vi "Write Next Trace ID.vi"(8 "error in (no error)":errorcluster, 10 "Next Trace ID":u64, 11 "Trace Controller in":refnum<class "Trace Controller.lvclass">) -> (0 "error out":errorcluster, 3 "Trace Controller out":refnum<class "Trace Controller.lvclass">)   [LabVIEW 2014, in "Robot Actor Framework.lvlib" / "Trace.lvlib" / "Trace Controller.lvclass"]
uses:
  Trace Controller.lvclass
  Trace Controller.lvclass/Trace Controller.ctl
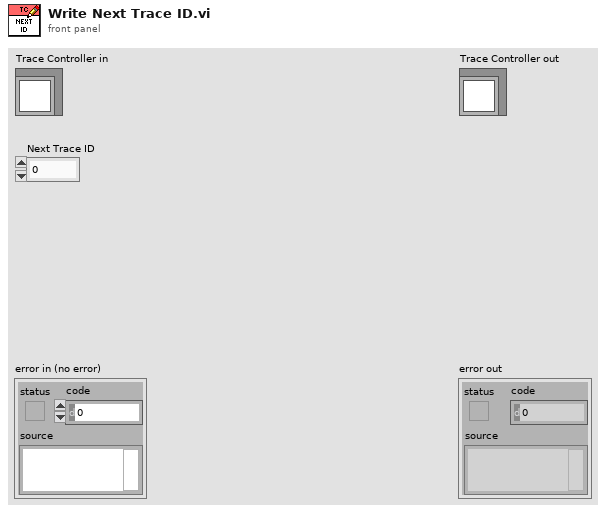
[diagram p1: front panel]
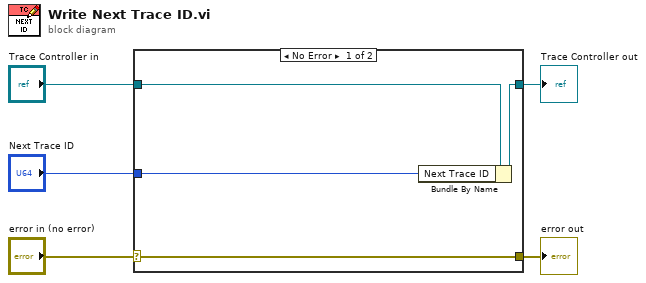
[diagram p0: block diagram]
diagram:
  n1 = case shown="No Error" "error in (no error)" {
    selector: "error in (no error)" -> [w9 w10]
    tunnel: [w9 w10] -> w4
    tunnel: [w7 w11] -> w2
    tunnel: "Trace Controller in" -> [w8 w11]
    tunnel: "Next Trace ID" -> [w6 _]
    frame No Error {
      n2 = Bundle By Name(cluster=w8, "Next Trace ID"=w6) -> (w7:refnum<class "Trace Controller.lvclass">)
    }
    frame Error {
    }
  }
  "error out" <- w4
  "Trace Controller out" <- w2
